vi "Unflatten Value.vi"(8 "error in (no error)":errorcluster, 10 "Value":string, 11 "Boolean in":refnum<class "Path 1D.lvclass">) -> (0 "error out":errorcluster, 3 "Boolean out":refnum<class "Path 1D.lvclass">)   [LabVIEW 2017, in "Path 1D.lvclass"]
uses:
  <vilib>/gpm_packages/@cs/data-type-serializer/source/Path 1D/Path 1D.lvclass
  <vilib>/gpm_packages/@cs/data-type-serializer/source/Path 1D/Path 1D.lvclass/Path 1D.ctl
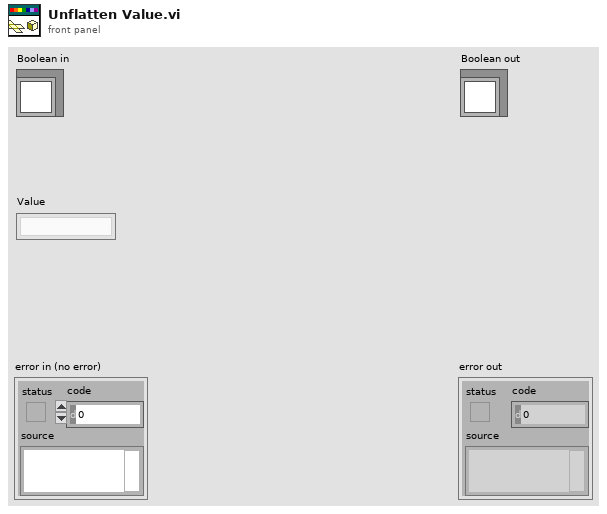
[diagram p1: front panel]
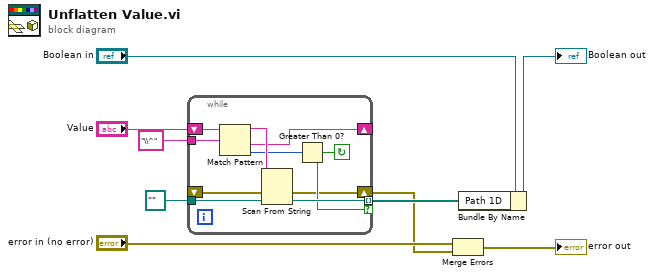
[diagram p0: block diagram]
diagram:
  n1 = while {
    tunnel: "\\^" ("regular expression") -> [w18]
    tunnel: path "" -> [w17]
    shift-right: [w15] -> _
    shift-left: "Value" -> [w19]
    tunnel: [w14] -> w2 mode=indexing if=w12
    shift-right: [w11] -> w1
    shift-left: _ -> [w10]
    stop <- w12 continue-if-true
    n2 = Match Pattern(string=w19, regular expression=w18) -> (before substring=w16:string, after substring=w15:string, offset past match=w13:i32)  [unwired: 1 in, 1 out]
    n3 = Scan From String(input string=w16, error in=w10, default 1=w17) -> (error out=w11:errorcluster, output 1=w14:path)  [unwired: 2 in, 2 out]
    n4 = Greater Than 0?(x=w13) -> (x > 0?=w12:bool)
  }
  n5 = Merge Errors("error in (no error)", w1) -> (→"error out":errorcluster)
  n6 = Bundle By Name(cluster="Boolean in", "Path 1D"=w2) -> (→"Boolean out":refnum<class "Path 1D.lvclass">)
